vi "brushless_motor_test.vi"() -> ()   [LabVIEW 2019]
uses:
  KNRm_ReMi_OS6_436Motor.lvlibp/KNRm_ReMi_Toolkit/IO/LowLevel/IOSETChannel.ctl
  KNRm_ReMi_OS6_436Motor.lvlibp/KNRm_ReMi_Toolkit/IO/LowLevel/IO_Channel_DIO.ctl
  KNRm_ReMi_OS6_436Motor.lvlibp
panel:
  in  "button":bool
  in  "stop":bool
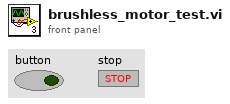
[diagram p1: front panel]
types:
  T1 = typedef "KNRm_ReMi_OS6_436Motor.lvlibp/IO_Channel_DIO.ctl" = enum16{"B/DIO1 (M1)", "A/DIO8 (M2)", "B/DIO7 (M3)", "A/DIO3 (M4)", "A/DIO14 (RC1_0)", "A/DIO15 (RC1_1)", "A/DIO7(S1)", "A/DIO2(S2)", "A/DIO6(S3)", "A/DIO3(S4)", "A/DIO5(S5)", "A/DIO4(S6)"}
  T2 = typedef "KNRm_ReMi_OS6_436Motor.lvlibp/IOSETChannel.ctl" = enum8{"0:B_DIO1/M1.EN/SM6.PULSE.CH1", "1:A_DIO8/M2.EN/SM6.DIR.CH1", "2:B_DIO7/M3.EN/SM6.PULSE.CH2", "3:A_DIO3/M4.EN/SM6.DIR.CH2", "4:A_DIO14/RC1_0", "5:A_DIO15/RC1_1", "6:LED(4)"}
  T3 = cluster{T2, "Checkbox":bool, "CycleTick":fxp<+,22,22>, "DutyCycleTick":fxp<+,22,22>}[]
  T4 = cluster{T2, "Checkbox":bool, "CycleTick":fxp<+,22,22>, "DutyCycleTick":fxp<+,22,22>}
  T5 = cluster{T2, "Checkbox":bool, "CycleTick":fxp<+,22,22>, "f":fxp<+,22,22>}
  T6 = cluster{T2, "Checkbox":bool, "CycleTick":fxp<+,22,22>, "f":fxp<+,22,22>}[]
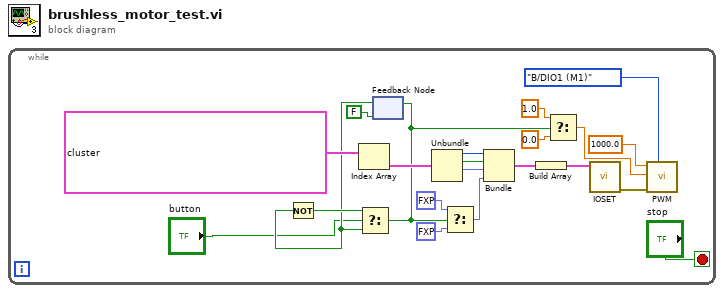
[diagram p0: block diagram]
diagram:
  n1 = while {
    stop <- "stop" stop-if-true
    n2 = Index Array(array=T3 [{enum."0:B_DIO1/M1.EN/SM6.PULSE.CH1", "Checkbox"=TRUE, "CycleTick"=0.0, "DutyCycleTick"=0.0}] ("IOSET")) -> (element=w21:T4)  [unwired: 1 in]
    n3 = feedback #1(FALSE ("F710 button info.Y")) -> (w2:bool)
    n4 = Not(x=w2) -> (.not. x?=w14:bool)
    n5 = Select(t=w14, s="button", f=w2) -> (s? t:f=w8:bool)
    n6 = feedback-in #1(w8) -> ()
    n7 = Unbundle(w21) -> (w20:T2, "Checkbox"=w19:bool, "CycleTick"=w18:fxp<+,22,22>)  [unwired: 1 out]
    n8 = Select(t=fxp<+,22,22> 1.0, s=w8, f=fxp<+,22,22> 0.0) -> (s? t:f=w11:fxp<+,22,22>)
    n9 = Bundle(w20, "Checkbox"=w19, "CycleTick"=w18, "f"=w11) -> (w17:T5)  [unwired: 1 in]
    n10 = Build Array(w17) -> (w16:T6)
    n11 = Select(t=1.0 ("DutyCycle"), s=w8, f=0.0 ("DutyCycle")) -> (s? t:f=w5:dbl)
    n12 = call "IOSET.vi"("IOSET"=w16) -> ("error out"=w4:errorcluster)  [unwired: 9 in, 1 out]
    n13 = call "PWM.vi"("IO_Chanel"=IO_Channel_DIO."B/DIO1 (M1)", "error in"=w4, "DutyCycle"=w5, "Frequency(Hz)"=1000.0) -> ()  [unwired: 7 in, 1 out]
  }
